vi "Reduce.vi"(8 "error in (no error)":errorcluster, 11 "SnailNum in":refnum<class "SnailNum.lvclass">) -> (0 "error out":errorcluster, 3 "SnailNum out":refnum<class "SnailNum.lvclass">)   [LabVIEW 2020, in "SnailNum.lvclass"]
uses:
  SnailNum.lvclass
  SnailNum.lvclass/SnailNum.ctl
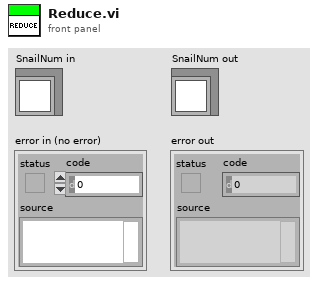
[diagram p1: front panel]
types:
  T1 = typedef "SnailNum.lvclass/Explode Result.ctl" = cluster{"Explode":bool, "Left Value":i64, "Right Value":i64, "Left Done":bool, "Right Done":bool}
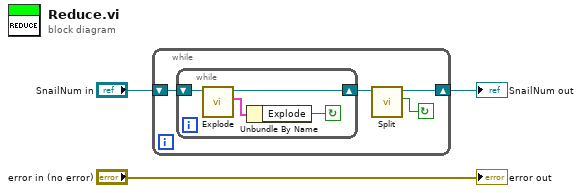
[diagram p0: block diagram]
diagram:
  n1 = while {
    shift-right: [w5] -> w1
    shift-left: "SnailNum in" -> [w7]
    stop <- w4 continue-if-true
    n2 = while {
      shift-right: [w8] -> w6
      shift-left: w7 -> [w11]
      stop <- w9 continue-if-true
      n3 = call "Explode.vi"("SnailNum in"=w11) -> ("Explode Result"=w10:T1, "SnailNum out"=w8:refnum<class "SnailNum.lvclass">)  [unwired: 8 in, 1 out]
      n4 = Unbundle By Name(w10) -> ("Explode"=w9:bool)
    }
    n5 = call "Split.vi"("SnailNum in"=w6) -> ("Did Split?"=w4:bool, "SnailNum out"=w5:refnum<class "SnailNum.lvclass">)  [unwired: 8 in, 1 out]
  }
  "SnailNum out" <- w1
  "error out" <- "error in (no error)"
